vi "svx_Convert Z Physical Units to Z Plot Index.vi"(5 "Z length":i32, 7 "Z Index":i32, 8 "Display State In":T2={"X Scale Width %"=50.0, "Y Scale Height %"=50.0, "X-Axis Range"={"Minimum"=0.0, "Maximum"=10.0}, "Y-Axis Range"={"Minimum"=0.0, "Maximum"=10.0}, "Z-Axis Range"={"Minimum"=0.0, "Maximum"=10.0}, "Plot Color"=61212, "Frame Color"=16252785, "Background Color"=16777222, "Initial AutoScale Y"=TRUE, "AutoScale X"=2, "AutoScale Y"=2, "AutoScale Z"=2, "Plot Transparency"=FALSE, "X-Axis Name"="Frequency", "Y-Axis Name"="Amplitude", "Z-Axis Name"="", "X-Axis Scaling Factor"={"Offset"=0.0, "Multiplier"=1.0}, "Y-Axis Scaling Factor"={"Offset"=0.0, "Multiplier"=1.0}, "Z-Axis Scaling Factor"={"Offset"=0.0, "Multiplier"=1.0}, "X-Scale Visible"=TRUE, "Y-Scale Visible"=TRUE, "Z-Scale Visible"=TRUE, "X-Scale Label Visible"=TRUE, "Y-Scale Label Visible"=TRUE, "Z-Scale Label Visible"=TRUE, "X-Axis Range Scaled"={"Minimum"=0.0, "Maximum"=10.0}, "Y-Axis Range Scaled"={"Minimum"=0.0, "Maximum"=10.0}, "Z-Axis Range Scaled"={"Minimum"=0.0, "Maximum"=10.0}, "Rev Z Order"=FALSE, "X-Scale Format Str"="%#.4g", "Y-Scale Format Str"="%#.4g", "Z-Scale Format Str"="%#.4g", "Decor color"=12369084, "Scale Range Change"=refnum, "out of state queue"=refnum, "property nodes"=refnum, "Lines"=[], "Line Properties"={"Line Color"=61212, "Line Width"=61212, "Line Style"=enum."Dash", "DisplayLines"=FALSE}} {"Line Properties"."Line Width" min=1}, 9 "z0":dbl, 10 "dz":dbl) -> (3 "Lines":T1[](array[typedef]))   [LabVIEW 2017, in "SVX Waterfall Graph.xctl"]
uses:
  <vilib>/addons/_XControls/Waterfall Graph/SVX Waterfall Graph.xctl
  <vilib>/addons/_XControls/Waterfall Graph/subVIs/svx_Waterfall State.ctl
  <vilib>/addons/_NISVFA/_Shared subVIs/Controls/svc_Cluster of Array of Cluster of XYZ.ctl
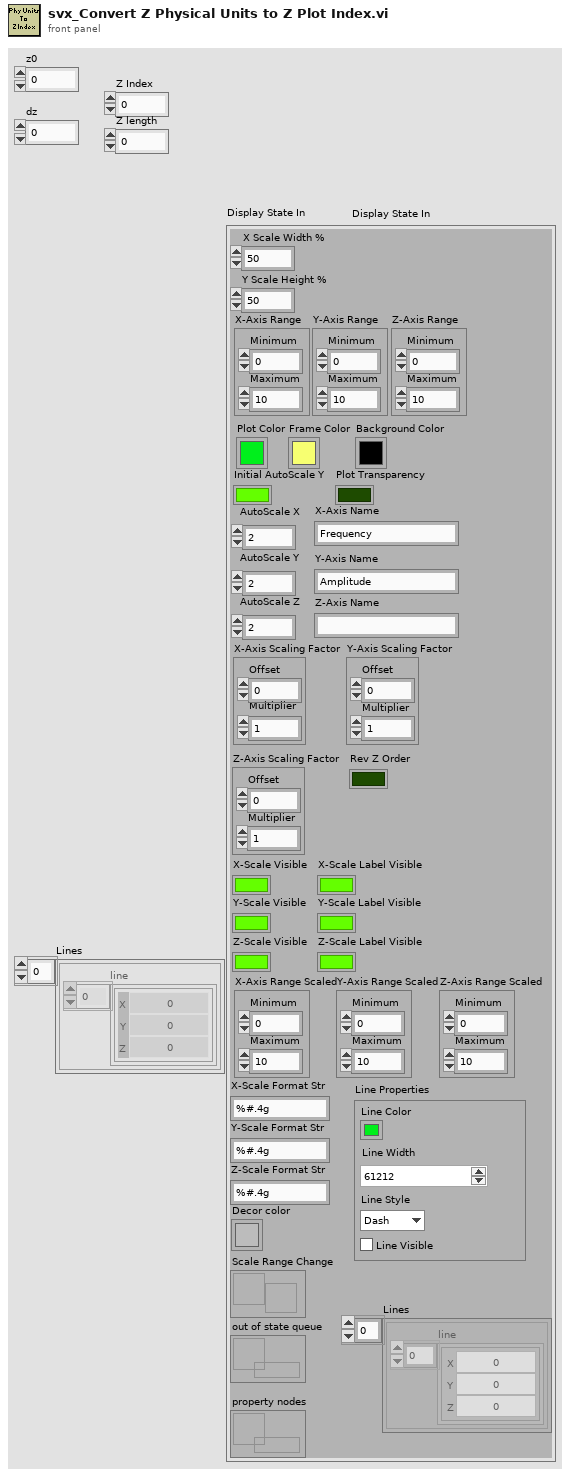
[diagram p1: front panel]
types:
  T1 = typedef "svc_Cluster of Array of Cluster of XYZ.ctl" = cluster{"line":cluster{"X":dbl, "Y":dbl, "Z":dbl}[]}
  T2 = typedef "SVX Waterfall Graph.xctl/svx_Waterfall State.ctl" = cluster{"X Scale Width %":dbl, "Y Scale Height %":dbl, "X-Axis Range":cluster{"Minimum":dbl, "Maximum":dbl}, "Y-Axis Range":cluster{"Minimum":dbl, "Maximum":dbl}, "Z-Axis Range":cluster{"Minimum":dbl, "Maximum":dbl}, "Plot Color":u32, "Frame Color":u32, "Background Color":u32, "Initial AutoScale Y":bool, "AutoScale X":u8, "AutoScale Y":u8, "AutoScale Z":u8, "Plot Transparency":bool, "X-Axis Name":string, "Y-Axis Name":string, "Z-Axis Name":string, "X-Axis Scaling Factor":cluster{"Offset":dbl, "Multiplier":dbl}, "Y-Axis Scaling Factor":cluster{"Offset":dbl, "Multiplier":dbl}, "Z-Axis Scaling Factor":cluster{"Offset":dbl, "Multiplier":dbl}, "X-Scale Visible":bool, "Y-Scale Visible":bool, "Z-Scale Visible":bool, "X-Scale Label Visible":bool, "Y-Scale Label Visible":bool, "Z-Scale Label Visible":bool, "X-Axis Range Scaled":cluster{"Minimum":dbl, "Maximum":dbl}, "Y-Axis Range Scaled":cluster{"Minimum":dbl, "Maximum":dbl}, "Z-Axis Range Scaled":cluster{"Minimum":dbl, "Maximum":dbl}, "Rev Z Order":bool, "X-Scale Format Str":string, "Y-Scale Format Str":string, "Z-Scale Format Str":string, "Decor color":u32, "Scale Range Change":refnum<user-event>, "out of state queue":refnum<queue>, "property nodes":refnum<queue>, "Lines":T1[], "Line Properties":cluster{"Line Color":u32, "Line Width":u16, "Line Style":enum32{"Solid", "Dash", "Dot", "DashDot", "DashDotDot"}, "DisplayLines":bool}}
  T3 = enum16{"Round To Nearest", "Round To -Inf", "Round to + Inf"}
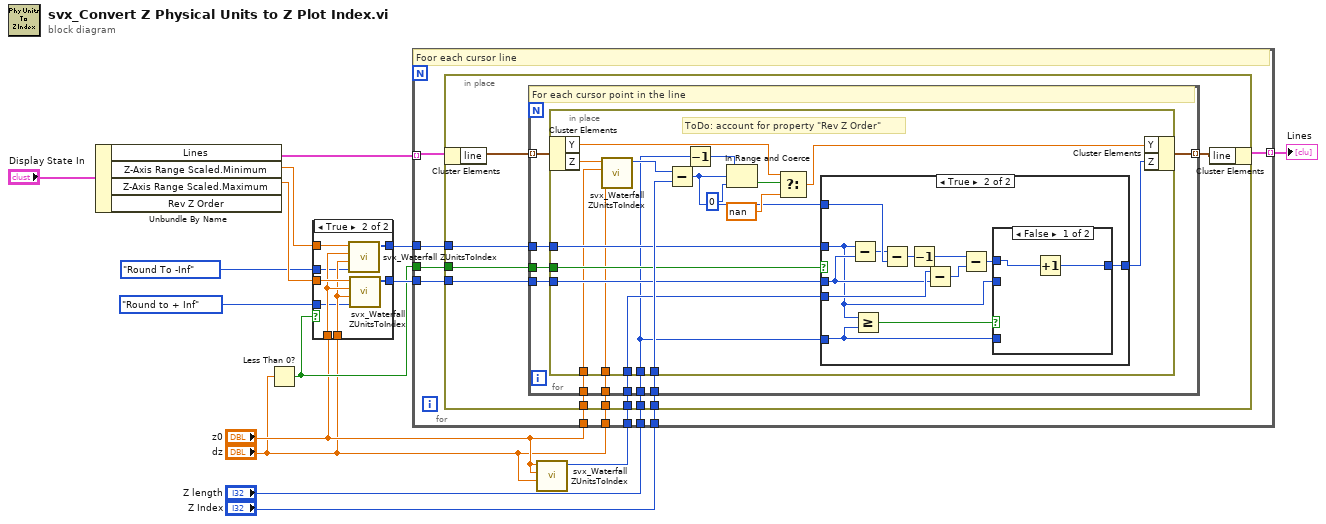
[diagram p0: block diagram]
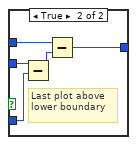
[diagram p4: hidden frame]
diagram:
  n1 = Unbundle By Name("Display State In") -> ("Lines"=w6:T1[], "Z-Axis Range Scaled.Minimum"=w7:dbl, "Z-Axis Range Scaled.Maximum"=w8:dbl)  [unwired: 1 out]
  n2 = Less Than 0?(x="dz") -> (x < 0?=w10:bool)
  n3 = case shown="True" w10 {
    tunnel: w7 -> [_ w23]
    tunnel: w8 -> [_ w22]
    tunnel: "z0" -> [_ w21]
    tunnel: [_ w20] -> w12
    tunnel: [_ w19] -> w11
    tunnel: "dz" -> [_ w18]
    tunnel: T3."Round To -Inf" ("Rounding Type") -> [_ w17]
    tunnel: T3."Round to + Inf" ("Rounding Type") -> [_ w16]
    frame False {
    }
    frame True {
      n4 = call <vilib>:"svx_Waterfall ZUnitsToIndex.vi"("Rounding Type"=w17, "dz"=w18, "z0"=w21, "Z In Units"=w23) -> ("ZIndex"=w20:i32)  [unwired: 7 in]
      n5 = call <vilib>:"svx_Waterfall ZUnitsToIndex.vi"("Rounding Type"=w16, "dz"=w18, "z0"=w21, "Z In Units"=w22) -> ("ZIndex"=w19:i32)  [unwired: 7 in]
    }
  }
  n6 = call <vilib>:"svx_Waterfall ZUnitsToIndex.vi"("dz"="dz", "z0"="z0", "Z In Units"="z0") -> ("ZIndex"=w1:i32)  [unwired: 8 in]
  n7 = for {
    tunnel: w6 -> [w25] mode=indexing
    tunnel: "z0" -> [w33]
    tunnel: "dz" -> [w32]
    tunnel: [w31] -> w9 mode=indexing
    tunnel: "Z Index" -> [w30]
    tunnel: "Z length" -> [w29]
    tunnel: w12 -> [w28]
    tunnel: w11 -> [w27]
    tunnel: w10 -> [w26]
    tunnel: w1 -> [w24]
    # "Foor each cursor line"
    n8 = in-place {
      in-place-border: w33 -> [w37]
      in-place-border: w32 -> [w36]
      in-place-border: w30 -> [w42]
      in-place-border: w29 -> [w35]
      in-place-border: w28 -> [w41]
      in-place-border: w27 -> [w40]
      in-place-border: w26 -> [w39]
      in-place-border: w24 -> [w34]
      n9 = in-place-cluster #1(w25) -> ("line"=w38:cluster{"X":dbl, "Y":dbl, "Z":dbl}[])
      n10 = for {
        tunnel: w38 -> [w51] mode=indexing
        tunnel: w37 -> [w53]
        tunnel: w36 -> [w52]
        tunnel: [w50] -> w43 mode=indexing
        tunnel: w42 -> [w49]
        tunnel: w35 -> [w48]
        tunnel: w41 -> [w47]
        tunnel: w40 -> [w46]
        tunnel: w39 -> [w45]
        tunnel: w34 -> [w44]
        # "For each cursor point in the line"
        n11 = in-place {
          in-place-border: w53 -> [w57]
          in-place-border: w52 -> [w58]
          in-place-border: w49 -> [w67]
          in-place-border: w48 -> [w54]
          in-place-border: w47 -> [w63]
          in-place-border: w46 -> [w62]
          in-place-border: w45 -> [w59]
          in-place-border: w44 -> [w55]
          # "ToDo: account for property \"Rev Z Order\""
          n12 = in-place-cluster #2(w51) -> ("Y"=w68:dbl, "Z"=w61:dbl)
          n13 = call <vilib>:"svx_Waterfall ZUnitsToIndex.vi"("dz"=w58, "z0"=w57, "Z In Units"=w61) -> ("ZIndex"=w60:i32)  [unwired: 8 in]
          n14 = Subtract(x=w60, y=w67) -> (x-y=w65:i32)
          n15 = Decrement(x=w54) -> (x-1=w56:i32)
          n16 = In Range and Coerce(upper limit=w56, x=w65, lower limit=0) -> (In Range?=w70:bool)  [unwired: 1 out]
          n17 = Select(t=w68, s=w70, f=nan ("Z")) -> (s? t:f=w66:dbl)
          n18 = case shown="True" w59 {
            tunnel: w65 -> [w72 w84]
            tunnel: [w72 w77] -> w64
            tunnel: w63 -> [_ w76]
            tunnel: w62 -> [_ w81]
            tunnel: w55 -> [_ w82]
            tunnel: w54 -> [_ w75]
            frame False {
            }
            frame True {
              n19 = Subtract(x=w76, y=w81) -> (x-y=w74:i32)
              n20 = Greater Or Equal?(x=w76, y=w75) -> (x >= y?=w79:bool)
              n21 = Subtract(x=w74, y=w84) -> (x-y=w83:i32)
              n22 = Decrement(x=w83) -> (x-1=w80:i32)
              n23 = Subtract(x=w82, y=w81) -> (x-y=w73:i32)
              n24 = Subtract(x=w80, y=w73) -> (x-y=w78:i32)
              n25 = case shown="False" w79 {
                tunnel: w78 -> [w86 w91]
                tunnel: [w85 w90] -> w77
                tunnel: w76 -> [_ w89]
                tunnel: w75 -> [_ w88]
                frame False {
                  n26 = Increment(x=w86) -> (x+1=w85:i32)
                }
                frame True {
                  # "Last plot above\nlower boundary"
                  n27 = Subtract(x=w89, y=w88) -> (x-y=w87:i32)
                  n28 = Subtract(x=w91, y=w87) -> (x-y=w90:i32)
                }
              }
            }
          }
          n29 = in-place-cluster #2("Y"=w66, "Z"=w64) -> (w50:cluster{"X":dbl, "Y":dbl, "Z":dbl})
        }
      }
      n30 = in-place-cluster #1("line"=w43) -> (w31:T1)
    }
  }
  "Lines" <- w9
